vi "Integrator Start-Stop.vi"(8 "error in (no error)":errorcluster, 9 "Start/Stop (F: Stop)":bool, 10 "Element (All: 0)":T1(ring), 11 "Yokogawa WT1600 in":refnum<class "Yokogawa WT1600.lvclass">) -> (0 "error out":errorcluster, 2 "VISA session":refnum<visa-resource-name>, 3 "Yokogawa WT1600 out":refnum<class "Yokogawa WT1600.lvclass">)   [LabVIEW 2013, in "Generic Power Analyzer.lvlib" / "Yokogawa WT1600.lvlib" / "Yokogawa WT1600.lvclass"]
uses:
  Yokogawa WT1600.lvclass
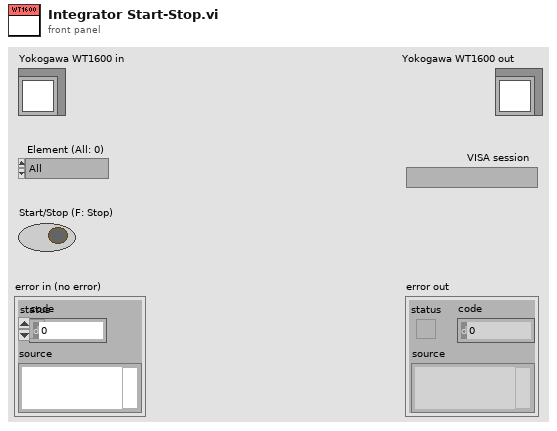
[diagram p1: front panel]
types:
  T1 = enum16{"All", "Element 1", "Element 2", "Element 3", "Element 4", "Element 5", "Element 6"}
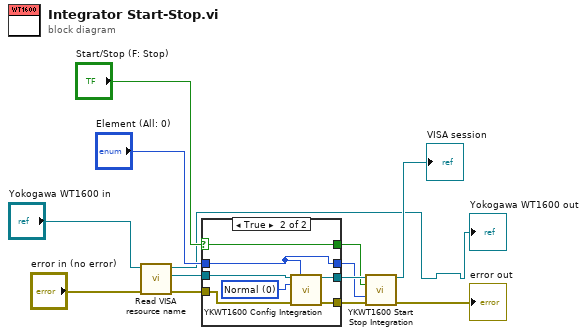
[diagram p0: block diagram]
diagram:
  n1 = call-dynamic "Read VISA resource name.vi"("error in (no error)"="error in (no error)", "Generic Instrument in"="Yokogawa WT1600 in") -> ("error out"=w5:errorcluster, "VISA resource name"=w7:refnum<visa-resource-name>, "Generic Instrument out"=→"Yokogawa WT1600 out":refnum<class "Yokogawa WT1600.lvclass">)  [unwired: 7 in]
  n2 = case shown="True" "Start/Stop (F: Stop)" {
    selector: "Start/Stop (F: Stop)" -> [w15 w19]
    tunnel: w7 -> [w17 w21]
    tunnel: w5 -> [w16 w23]
    tunnel: [w16 w22] -> w10
    tunnel: [w17 w20] -> w11
    tunnel: "Element (All: 0)" -> [w14 w18]
    tunnel: [w15 w19] -> w4
    tunnel: [w14 w18] -> w3
    frame False {
    }
    frame True {
      w24 = u16 0 items=["Normal", "Continuous"] ("Integ Mode (0: Normal)")
      n3 = call <instrlib>:"YKWT1600 Config Integration.vi"("VISA session"=w21, "Element (0: All)"=w18, "Integ Mode (0: Normal)"=w24, "error in (no error)"=w23) -> ("dup VISA session"=w20:refnum<visa-resource-name>, "error out"=w22:errorcluster)  [unwired: 10 in]
    }
  }
  n4 = call <instrlib>:"YKWT1600 Start Stop Integration.vi"("VISA session"=w11, "Start/Stop (F: Stop)"=w4, "Element (All: 0)"=w3, "error in (no error)"=w10) -> ("dup VISA session"=→"VISA session":refnum<visa-resource-name>, "error out"=→"error out":errorcluster)  [unwired: 10 in]
